vi "Shooter Loop.vi"   [LabVIEW 2015]
uses:
  Common Code/Shooter State.ctl
  Robot Global Data.vi
types:
  T1 = typedef "Shooter Command Cluster.ctl" = cluster{"Command":T2, "Mode":T3, "Shot Type":T4, "Override Trigger IR":bool, "Override Angle?":bool}
  T2 = typedef "Shooter Commands.ctl" = enum16{"Idle", "Prime Shooter", "Shoot"}
  T3 = typedef "Shoot Modes Enum.ctl" = enum16{"Manual", "Safe", "Auto"}
  T4 = typedef "Shot Type.ctl" = enum16{"Batter Shot", "Corner Shot", "Curve Shot", "Vision Shot", "Deep Middle Shot"}
  T5 = typedef "Manual Shoot.ctl" = cluster{"Spin Wheels":bool, "Fire":bool, "Angle":dbl, "Angle Power":dbl, "Use Manual Angle":bool, "Override RPM":bool, "Left RPM":dbl, "Right RPM":dbl, "Secure Ball?":bool}
  T6 = typedef "WPI_DigitalInputDevRef.ctl" = cluster{"DevStatus":errorcluster, "DIO Channel":T7}
  T7 = typedef "FPGA_DIOChannel.ctl" = enum8{"DIO 0", "DIO 1", "DIO 2", "DIO 3", "DIO 4", "DIO 5", "DIO 6", "DIO 7", "DIO 8", "DIO 9", "DIO MXP 0", "DIO MXP 1", "DIO MXP 2", "DIO MXP 3", "DIO MXP 4", "DIO MXP 5", "DIO MXP 6", "DIO MXP 7", "DIO MXP 8", "DIO MXP 9", "DIO MXP 10", "DIO MXP 11", "DIO MXP 12", "DIO MXP 13", "DIO MXP 14", "DIO MXP 15", "Invalid"}
  T8 = typedef "Dashboard Control Data.ctl" = cluster{"Encoder Control":T9, "Steer PID output":cluster{"output high":dbl, "output low":dbl}, " Steer PID gains":cluster{"proportional gain (Kc)":dbl, "integral time (Ti, min)":dbl, "derivative time (Td, min)":dbl}, "Drivetrain Settings":T10, "Vision Packet":T11, "Info/Command Cluster":T12, "Ball Vision Packet":T13, "Intake Presets":T15, "Intake Encoder Control":T17, "Climb Presets":T18, "Goal Output Range":cluster{"output high":dbl, "output low":dbl}, "Shooter Presets":T19}
  T9 = typedef "Encoder Control.ctl" = cluster{"Right Tick Constant":dbl, "Left Tick Constant":dbl, "Reset?":bool, "Y Dist":cluster{"PID gains":cluster{"proportional gain (Kc)":dbl, "integral time (Ti, min)":dbl, "derivative time (Td, min)":dbl}}, "Y Stop Thresh":dbl, "Y Stop Speed":dbl}
  T10 = typedef "Drivetrain Settings.ctl" = cluster{"Gyro Tolerance":dbl, "Throttle Ramp (ms)":dbl, "Angular rate compensation":bool, "Throttle to Rate Scale":dbl, "Rate compensation gain":dbl, "Kv":dbl, "Ka":dbl, "Feed Forward P":dbl, "Feed Forward D":dbl, "Goal Vision PID gains":cluster{"proportional gain (Kc)":dbl, "integral time (Ti, min)":dbl, "derivative time (Td, min)":dbl}, "Goal Detection Window":dbl}
  T11 = typedef "Goal Vision Packet.ctl" = cluster{"Distance":dbl, "Center X":dbl, "Center Y":dbl, "Found Target?":bool}
  T12 = typedef "Ball Tracking Command Cluster.ctl" = cluster{"Distance to Ball":dbl, "Desired Angle":dbl, "Command":enum16{"Turn to Ball", "Turn to Angle", "Get Distance"}, "Pixels from Center":dbl}
  T13 = typedef "Ball Vision Packet.ctl" = cluster{"Ball Detected?":bool, "Distance to Ball":dbl, "Desired Angle":dbl, "Pixels from Center":dbl, "Tracking mode":T14}
  T14 = typedef "Tracking Mode.ctl" = enum16{"Turn to Ball", "Turn to Angle"}
  T15 = typedef "Intake Presets.ctl" = cluster{"Intake Speed":dbl, "Outake Speed":dbl, "Low Height":dbl, "Half Height":dbl, "Full Height":dbl, "Angle Speed":dbl, "Fast Angle":dbl, "Encoder Scale":dbl, "Load Height":dbl, "Output Range":T16, "Rotation Power Max/Min":dbl, "MaxCurrent":dbl, "Intake Trip Time":dbl, "Idle Height":dbl, "Max Height":dbl, "Reset Encoders?":bool, "PID gains":cluster{"proportional gain (Kc)":dbl, "integral time (Ti, min)":dbl, "derivative time (Td, min)":dbl}}
  T16 = typedef "Drivetrain Output Range.ctl" = cluster{"output high":dbl, "output low":dbl}
  T17 = typedef "IntakeEcoderControl.ctl" = cluster{"Arm Tick Constant":dbl, "Reset?":bool, "Y Dist":cluster{"PID gains":cluster{"proportional gain (Kc)":dbl, "integral time (Ti, min)":dbl, "derivative time (Td, min)":dbl}}, "Y Stop Thresh":dbl, "Y Stop Speed":dbl}
  T18 = typedef "Climb Presets.ctl" = cluster{"Pull Power":dbl, "Unpin Power":dbl, "Time to Hold":dbl}
  T19 = typedef "Shooter Presets.ctl" = cluster{"Batter Shot":T20, "Deep Middle Shot":T20, "Manual Shot":T20, "Left Ticks Per Rotation":dbl, "Right Ticks Per Rotation":dbl, "Low Bar Shot":T20, "Shooter RPM Tolerance":dbl, "IIR Filter Power":dbl, "Trigger Power":dbl, "Fire from Load Delay":i32, "Angle Pot M":dbl, "Angle Pot B":dbl, "Shooter Length":dbl, "String Pot Dist":dbl, "Angle PID gains":cluster{"proportional gain (Kc)":dbl, "integral time (Ti, min)":dbl, "derivative time (Td, min)":dbl}, "Angle Motor Output":cluster{"output high":dbl, "output low":dbl}, "Shooter Angle Tolerance":dbl, "Vision Shoot x^2":dbl, "Vision Shoot x":dbl, "Dist from Axis Cam to Pivot":dbl, "High Goal Center Height":dbl, "Feed Forward Max Accel":dbl, "Feed Forward Kv":dbl, "Backwards Trigger":dbl, "Shot Finish Delay (ms)":dbl, "Angle Max Current":dbl, "Angle Current Trip Time":dbl, "Shooter Intake Angle":dbl, "Vision Shoot c":dbl, "Reset?":bool, "Servo Release Delay":dbl, "Servo Idle Angle":i32, "Servo Hold Angle":i32, "Angle Pot x^2":dbl, "Angle Pot x":dbl, "Angle Pot c":dbl}
  T20 = typedef "Shot Presets.ctl" = cluster{"Left Wheel RPM":dbl, "Right Wheel RPM":dbl, "Angle":dbl}
  T21 = typedef "Shooter State.ctl" = enum16{"Idle", "Warmup", "Shooter Ready", "Shoot"}
  T22 = typedef "WPI_ServoDeviceRef.ctl" = cluster{"DeviceStatus":errorcluster, "PWM Channel":T23, "DeadBand":T24}
  T23 = typedef "FPGA_DIOPWMChannel.ctl" = enum8{"PWM 0", "PWM 1", "PWM 2", "PWM 3", "PWM 4", "PWM 5", "PWM 6", "PWM 7", "PWM 8", "PWM 9", "PWM MXP 0", "PWM MXP 1", "PWM MXP 2", "PWM MXP 3", "PWM MXP 4", "PWM MXP 5", "PWM MXP 6", "PWM MXP 7", "PWM MXP 8", "PWM MXP 9", "Invalid"}
  T24 = typedef "WPI_PWMDeadband.ctl" = cluster{"Name":string, "maxPositivePwm":i32, "minPositivePwm":i32, "centerPwm":i32, "maxNegativePwm":i32, "minNegativePwm":i32, "angularRange":u16}
  T25 = typedef "WPI_MotorControlDeviceRef.ctl" = cluster{"DeviceStatus":errorcluster, "Type":T26, "PWM":cluster{"PWM Channel":T23, "DeadBand":T24}, "CAN":cluster{"Device Number":u8, "Control Mode":T27, "Semaphore":T28, "Max Vout":dbl, "TalonSRX Control Mode":T29}, "Invert":bool}
  T26 = typedef "WPI_MotorControlType.ctl" = enum16{"PWM", "CAN", "CANTalonSRX"}
  T27 = typedef "WPI_CANJaguar_ControlMode.ctl" = enum8{"Percent VBus", "Current", "Speed", "Position", "Voltage"}
  T28 = typedef "Semaphore RefNum" = refnum<k1>
  T29 = typedef "WPI_CANTalonSRX_APIControlMode.ctl" = enum8{"Percent VBus", "Speed", "Position", "Slave", "Unchanged / Invalid", "Voltage Compensation", "Current", "Motion Profile"}
  T30 = typedef "Shooter State Cluster.ctl" = cluster{"State":T21, "Left RPM":dbl, "Right RPM":dbl, "Shooter Ready?":bool, "Ball Loaded?":bool, "Current Angle":dbl, "Angle Motor Output":dbl, "Trigger Output":dbl, "Angle Ready?":bool, "RPM Ready?":bool, "Vision Ready?":bool, "Ball Loaded?":bool, "Mode":T3, "Shot Type":T4, "Pot Height":dbl, "Current Tripped Forward?":bool, "Current Tripped Backward?":bool, "Left Motor":dbl, "Right Motor":dbl, "Intake High?":bool, "Raw Left Pos":dbl, "Raw Right Pos":dbl, "Raw Left V":dbl, "Raw Right V":dbl, "Right Servo":i32, "Left Servo":i32}
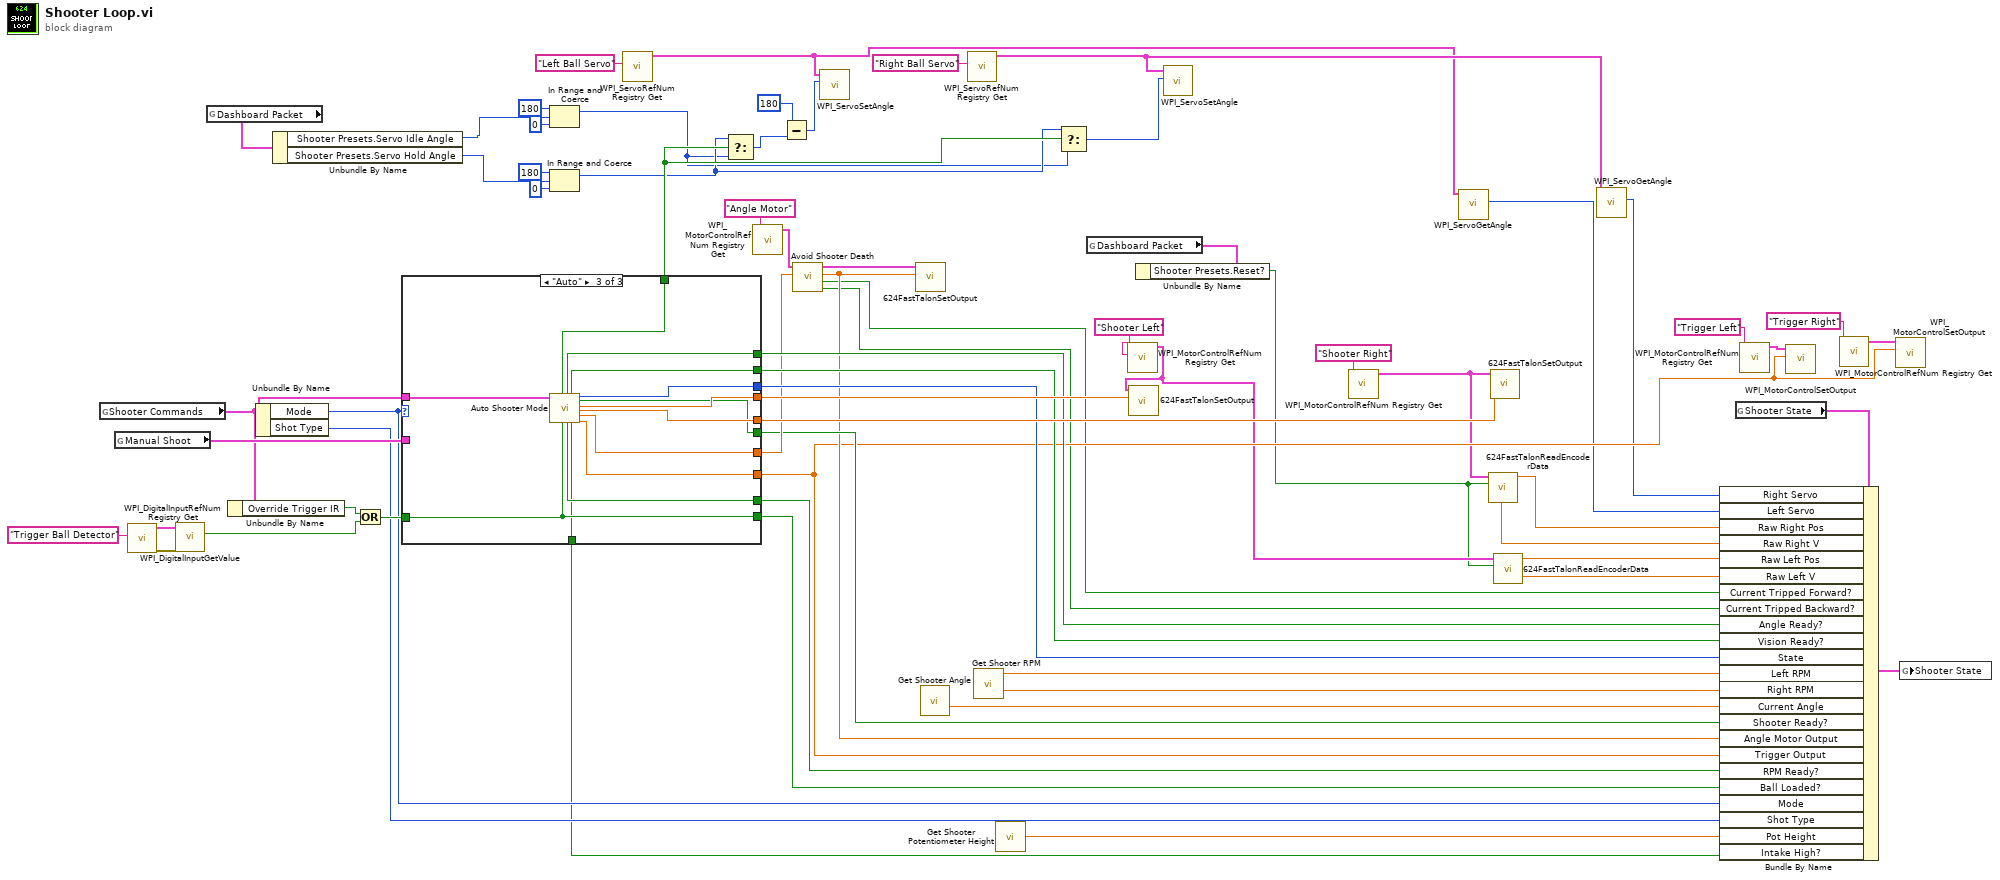
[diagram p0: block diagram]
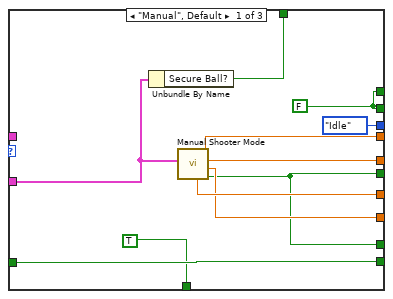
[diagram p2: hidden frame]
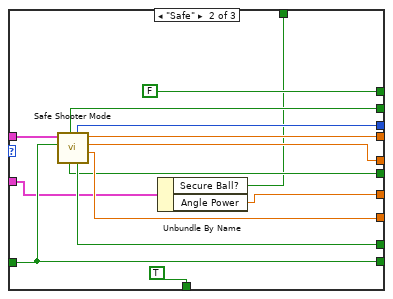
[diagram p3: hidden frame]
diagram:
  n1 = global read "Robot Global Data.vi" "Shooter Commands"() -> (w57:T1)
  n2 = global read "Robot Global Data.vi" "Manual Shoot"() -> (w65:T5)
  n3 = call <vilib>:"WPI_DigitalInputRefNum Registry Get.vi"("refnum name"="Trigger Ball Detector") -> ("error out"=w60:errorcluster, "DigitalInputDevRef"=w59:T6)  [unwired: 9 in]
  n4 = call <vilib>:"WPI_DigitalInputGetValue.vi"("error in (no error)"=w60, "DigitalInputDevRef"=w59) -> ("Value"=w55:bool)  [unwired: 7 in, 2 out]
  n5 = global read "Robot Global Data.vi" "Dashboard Packet"() -> (w17:T8)
  n6 = Unbundle By Name(w57) -> ("Override Trigger IR"=w56:bool)
  n7 = Unbundle By Name(w57) -> ("Mode"=w47:T3, "Shot Type"=w46:T4)
  n8 = Unbundle By Name(w17) -> ("Shooter Presets.Servo Idle Angle"=w11:i32, "Shooter Presets.Servo Hold Angle"=w6:i32)
  n9 = Or(x=w56, y=w55) -> (x .or. y?=w54:bool)
  n10 = case shown="\"Auto\"" w47 {
    tunnel: w57 -> [_ w92 w105]
    tunnel: w65 -> [w69 w82 _]
    tunnel: [w78 w90 w99] -> w62
    tunnel: [w75 w89 w100] -> w61
    tunnel: [w73 w84 w95] -> w43
    tunnel: w54 -> [w77 w91 w104]
    tunnel: [w77 w91 w104] -> w51
    tunnel: [w76 w81 w101] -> w45
    tunnel: [w74 w88 w102] -> w33
    tunnel: [w73 w86 w103] -> w50
    tunnel: [Shooter_State."Idle" ("State") w87 w98] -> w52
    tunnel: [w71 w85 w97] -> w48
    tunnel: [w71 FALSE ("Angle In Range?") w96] -> w49
    tunnel: [TRUE ("Intake High Angle Allowed?") TRUE ("Intake High Angle Allowed?") w94] -> w38
    tunnel: [w68 w79 w93] -> w18
    frame "Manual", Default {
      w71 = FALSE ("Vision Target Aligned?")
      n11 = Unbundle By Name(w69) -> ("Secure Ball?"=w68:bool)
      n12 = call "Manual Shooter Mode.vi"("Manual Shoot"=w69) -> ("Shooter Ready?"=w73:bool, "Trigger Output"=w74:dbl, "Right Output"=w75:dbl, "Left Output"=w78:dbl, "Angle Motor Out"=w76:dbl)  [unwired: 6 in]
    }
    frame "Safe" {
      n13 = call "Safe Shooter Mode.vi"("Ball Detected?"=w91, "Shooter Commands"=w92) -> ("Trigger Power"=w88:dbl, "Right Power"=w89:dbl, "Left Power"=w90:dbl, "RPM Ready?"=w86:bool, "State"=w87:T21, "Shooter Ready?"=w84:bool, "Vision Ready?"=w85:bool)  [unwired: 3 in]
      n14 = Unbundle By Name(w82) -> ("Secure Ball?"=w79:bool, "Angle Power"=w81:dbl)
    }
    frame "Auto" {
      n15 = call "Auto Shooter Mode.vi"("Shooter Command"=w105, "Ball Loaded?"=w104) -> ("Secure Ball?"=w93:bool, "Angle In Range?"=w96:bool, "RPM Ready?"=w103:bool, "Vision Target Aligned?"=w97:bool, "Intake High Angle Allowed?"=w94:bool, "State"=w98:T21, "Shooter Ready?"=w95:bool, "Left Output"=w99:dbl, "Right Output"=w100:dbl, "Angle Motor Output"=w101:dbl, "Trigger Output"=w102:dbl)  [unwired: 7 in]
    }
  }
  n16 = In Range and Coerce(upper limit=180, x=w11, lower limit=0) -> (coerced(x)=w4:i32)  [unwired: 1 out]
  n17 = In Range and Coerce(upper limit=180, x=w6, lower limit=0) -> (coerced(x)=w5:i32)  [unwired: 1 out]
  n18 = call <vilib>:"WPI_ServoRefNum Registry Get.vi"("refnum name"="Left Ball Servo") -> ("ServoDeviceRef"=w13:T22)  [unwired: 9 in, 1 out]
  n19 = Select(t=w5, s=w18, f=w4) -> (s? t:f=w2:i32)
  n20 = call <vilib>:"WPI_MotorControlRefNum Registry Get.vi"("refnum name"="Angle Motor") -> ("MotorControlDevRef"=w44:T25)  [unwired: 9 in, 1 out]
  n21 = Subtract(x=180, y=w2) -> (x-y=w1:i32)
  n22 = call "Avoid Shooter Death.vi"("Proposed Power"=w45, "CAN Talon SRX Ref"=w44) -> ("Reverse Trip?"=w31:bool, "Forward Trip?"=w32:bool, "Actual Output"=w41:dbl, "CAN Talon SRX Ref 2"=w42:T25)  [unwired: 6 in]
  n23 = call <vilib>:"WPI_ServoSetAngle.vi"("Angle"=w1, "ServoDeviceRef"=w13) -> ()  [unwired: 8 in, 2 out]
  n24 = call "624FastTalonSetOutput.vi"("Output"=w41, "MotorControlDevRef"=w42) -> ()  [unwired: 8 in, 2 out]
  n25 = call "Get Shooter Angle.vi"() -> ("Current Angle"=w40:dbl)  [unwired: 11 in]
  n26 = call <vilib>:"WPI_ServoRefNum Registry Get.vi"("refnum name"="Right Ball Servo") -> ("ServoDeviceRef"=w16:T22)  [unwired: 9 in, 1 out]
  n27 = call "Get Shooter RPM.vi"() -> ("Right RPM"=w29:dbl, "Left RPM"=w30:dbl)  [unwired: 9 in, 1 out]
  n28 = call "Get Shooter Potentiometer Height.vi"() -> ("Height"=w39:dbl)  [unwired: 11 in]
  n29 = Select(t=w5, s=w18, f=w4) -> (s? t:f=w14:i32)
  n30 = global read "Robot Global Data.vi" "Dashboard Packet"() -> (w22:T8)
  n31 = call <vilib>:"WPI_MotorControlRefNum Registry Get.vi"("refnum name"="Shooter Left") -> ("MotorControlDevRef"=w25:T25)  [unwired: 9 in, 1 out]
  n32 = call "624FastTalonSetOutput.vi"("Output"=w62, "MotorControlDevRef"=w25) -> ()  [unwired: 8 in, 2 out]
  n33 = Unbundle By Name(w22) -> ("Shooter Presets.Reset?"=w21:bool)
  n34 = call <vilib>:"WPI_ServoSetAngle.vi"("Angle"=w14, "ServoDeviceRef"=w16) -> ()  [unwired: 8 in, 2 out]
  n35 = call <vilib>:"WPI_MotorControlRefNum Registry Get.vi"("refnum name"="Shooter Right") -> ("MotorControlDevRef"=w28:T25)  [unwired: 9 in, 1 out]
  n36 = call <vilib>:"WPI_ServoGetAngle.vi"("ServoDeviceRef"=w13) -> ("Angle"=w12:u16)  [unwired: 7 in, 2 out]
  n37 = call "624FastTalonReadEncoderData.vi"("Reset?"=w21, "CAN Talon SRX Ref"=w28) -> ("Encoder Velocity"=w26:dbl, "Encoder Position"=w27:dbl)  [unwired: 4 in, 4 out]
  n38 = call "624FastTalonSetOutput.vi"("Output"=w61, "MotorControlDevRef"=w28) -> ()  [unwired: 8 in, 2 out]
  n39 = call "624FastTalonReadEncoderData.vi"("Reset?"=w21, "CAN Talon SRX Ref"=w25) -> ("Encoder Velocity"=w23:dbl, "Encoder Position"=w24:dbl)  [unwired: 4 in, 4 out]
  n40 = call <vilib>:"WPI_ServoGetAngle.vi"("ServoDeviceRef"=w16) -> ("Angle"=w15:u16)  [unwired: 7 in, 2 out]
  n41 = global read "Robot Global Data.vi" "Shooter State"() -> (w67:T30)
  n42 = Bundle By Name(cluster=w67, "Right Servo"=w15, "Left Servo"=w12, "Raw Right Pos"=w27, "Raw Right V"=w26, "Raw Left Pos"=w24, "Raw Left V"=w23, "Current Tripped Forward?"=w32, "Current Tripped Backward?"=w31, "Angle Ready?"=w49, "Vision Ready?"=w48, "State"=w52, "Left RPM"=w30, "Right RPM"=w29, "Current Angle"=w40, "Shooter Ready?"=w43, "Angle Motor Output"=w41, "Trigger Output"=w33, "RPM Ready?"=w50, "Ball Loaded?"=w51, "Mode"=w47, "Shot Type"=w46, "Pot Height"=w39, "Intake High?"=w38) -> (w66:T30)
  n43 = call <vilib>:"WPI_MotorControlRefNum Registry Get.vi"("refnum name"="Trigger Left") -> ("MotorControlDevRef"=w35:T25)  [unwired: 9 in, 1 out]
  n44 = call <vilib>:"WPI_MotorControlSetOutput.vi"("Output"=w33, "MotorControlDevRef"=w35) -> ()  [unwired: 7 in, 3 out]
  n45 = call <vilib>:"WPI_MotorControlRefNum Registry Get.vi"("refnum name"="Trigger Right") -> ("MotorControlDevRef"=w34:T25)  [unwired: 9 in, 1 out]
  n46 = call <vilib>:"WPI_MotorControlSetOutput.vi"("Output"=w33, "MotorControlDevRef"=w34) -> ()  [unwired: 7 in, 3 out]
  n47 = global write "Robot Global Data.vi" "Shooter State"(w66) -> ()
